vi "Write to Waveform Log Instance.vi"(6 "tf Modified?":bool, 7 "Wfm Index":i32, 8 "error in (no error)":errorcluster, 9 "Data":dbl[](array[numeric]), 10 "Waveform Data":T5, 11 "Log Instance in":T1) -> (0 "error out":errorcluster, 3 "Log Instance out":T1)   [LabVIEW 2015, in "Waveform Log.lvclass"]
uses:
  Waveform Log.lvclass
  Log Instance.ctl
  Logs/Segmented Logs/Segmented Log/Segmented Log.lvclass
  Log Instance Waveform.ctl
  Waveform Information.ctl
  Waveform Data Type.ctl
  Waveform Log Wfm Meta Data.ctl
  Logs/Segmented Logs/Segmented Log/Segmented Log Waveform Meta Data.ctl
  Logs/Segmented Logs/Segmented Log/Segmented Log.lvclass/Segmented Log.ctl
  Log File Specifications/Log File Specification/Log File Specification.lvclass/Log File Specification.ctl
  Log File Specifications/Waveform TDMS Log File Specification/Waveform TDMS Log File Specification.lvclass/Waveform TDMS Log File Specification.ctl
  Logs/Log Files/Log File/Log File.lvclass/Log File.ctl
  Logs/Log Files/TDMS Log File/TDMS Log File.lvclass/TDMS Log File.ctl
  Logs/Log Files/Text Log File/Text Log File.lvclass/Text Log File.ctl
  Logs/Segmented Logs/Footprint Segmented Log/Footprint Segmented Log.lvclass/Footprint Segmented Log.ctl
  Logs/Segmented Logs/Time Segmented Log/Time Segmented Log.lvclass/Time Segmented Log.ctl
  Log File Specifications/Log File Specification/Get Log Specification Type.vi
  Log File Specifications/Waveform TDMS Log File Specification/Get Current Group.vi
  Logs/Log Files/Log File/Get Log File Type.vi
  Logs/Log Files/Log File/Write Channel to Log File.vi
  Logs/Log Files/TDMS Log File/Set TDMS Channel Property.vi
  Logs/Log Files/TDMS Log File/Copy Channel Properties.vi
  Logs/Segmented Logs/Segmented Log/Check Close File.vi
  Logs/Segmented Logs/Segmented Log/Check Open File.vi
  Logs/Log Files/TDMS Log File/Write Channel to TDMS Log File.vi
  Logs/Log Files/Text Log File/Write Channel to Text Log File.vi
  Logs/Segmented Logs/Segmented Log/Close Log File Instance.vi
  Logs/Segmented Logs/Segmented Log/Segment Log File.vi
  Logs/Segmented Logs/Segmented Log/Open Log File Instance.vi
  Logs/Log Files/Log File/Close Log File.vi
  Logs/Segmented Logs/Segmented Log/Make File Read-Only.vi
  Logs/Segmented Logs/Segmented Log/On Segmented Log Complete.vi
  Logs/Segmented Logs/Segmented Log/On File Close.vi
  Logs/Segmented Logs/Footprint Segmented Log/Segment Log File (Footprint).vi
  Logs/Segmented Logs/Time Segmented Log/Segment Log File (Time).vi
  Log File Specifications/Log File Specification/Open Log File.vi
  Log File Specifications/Log File Specification/Set Path Tag.vi
  Logs/Segmented Logs/Segmented Log/On File Open.vi
  Log File Specifications/Log File Specification/Set Filename Offset.vi
  Logs/Log Files/TDMS Log File/Close TDMS Log File.vi
  Logs/Log Files/Text Log File/Close Text Log File.vi
  Logs/Segmented Logs/Segmented Log/Get Current Log File Instance.vi
  Logs/Log Files/Log File/Get File Size.vi
  Logs/Log Files/Log File/Get Start Time.vi
  Log File Specifications/Log File Specification/Build File Path.vi
  Log File Specifications/Log File Specification/Resolve File Conflicts.vi
  Shared/Utility/Format File Path for Linux.vi
  <vilib>/Utility/error.llb/Error Cluster From Error Code.vi
  Log File Specifications/Log File Specification/Initialize Log File.vi
  <vilib>/Utility/libraryn.llb/Create Directory Recursive.vi
  <vilib>/Utility/libraryn.llb/Check if File or Folder Exists.vi
  <vilib>/Utility/libraryn.llb/Get File Extension.vi
  Logs/Log Files/Text Log File/Text Log File.lvclass
  Logs/Log Files/TDMS Log File/TDMS Log File.lvclass
  Logs/Log Files/Log File/Log File.lvclass
  Logs/Segmented Logs/Time Segmented Log/Time Segmented Log.lvclass
  Logs/Segmented Logs/Footprint Segmented Log/Footprint Segmented Log.lvclass
  Log File Specifications/Waveform TDMS Log File Specification/Waveform TDMS Log File Specification.lvclass
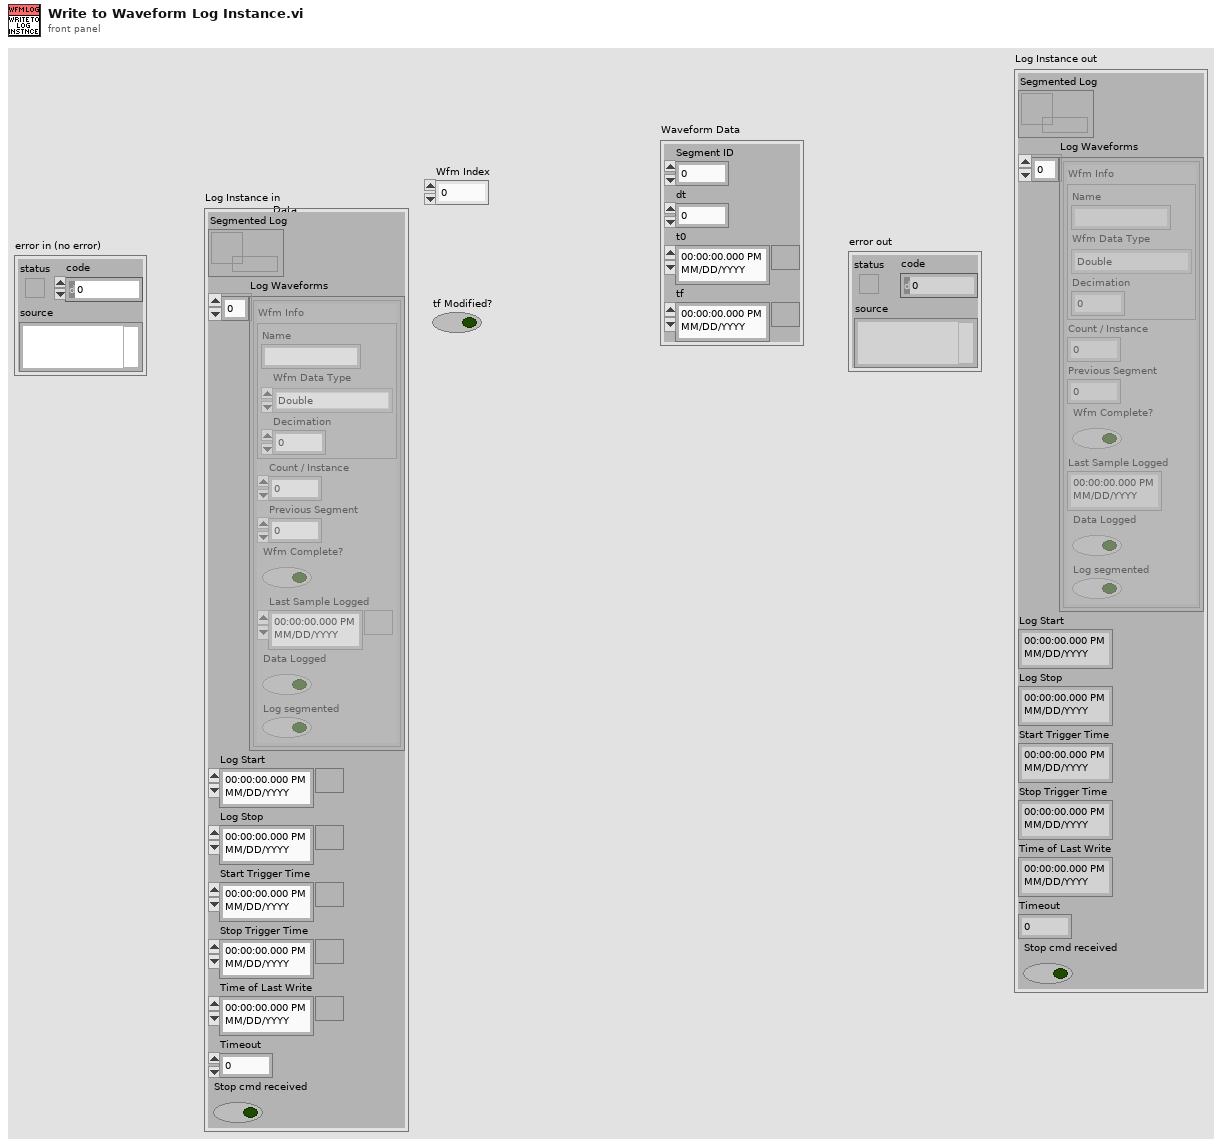
[diagram p1: front panel]
types:
  T1 = typedef "Waveform Log.lvclass/Log Instance.ctl" = cluster{"Segmented Log":refnum<data-value>, "Log Waveforms":T2[], "Log Start":timestamp, "Log Stop":timestamp, "Start Trigger Time":timestamp, "Stop Trigger Time":timestamp, "Time of Last Write":timestamp, "Timeout":dbl, "Stop cmd received":bool}
  T2 = typedef "Waveform Log.lvclass/Log Instance Waveform.ctl" = cluster{"Wfm Info":T3, "Count / Instance":i32, "Previous Segment":u64, "Wfm Complete?":bool, "Last Sample Logged":timestamp, "Data Logged":bool, "Log segmented":bool}
  T3 = typedef "Waveform Log.lvclass/Waveform Information.ctl" = cluster{"Name":string, "Wfm Data Type":T4, "Decimation":u32}
  T4 = typedef "Waveform Log.lvclass/Waveform Data Type.ctl" = enum16{"Double", "ComplexDouble"}
  T5 = typedef "Waveform Log.lvclass/Waveform Log Wfm Meta Data.ctl" = cluster{"Segment ID":u64, "dt":dbl, "t0":timestamp, "tf":timestamp}
  T6 = typedef "Segmented Log.lvclass/Segmented Log Waveform Meta Data.ctl" = cluster{"New Wfm Instance?":bool, "Wfm Instance":i32, "dt":dbl, "t0":timestamp}
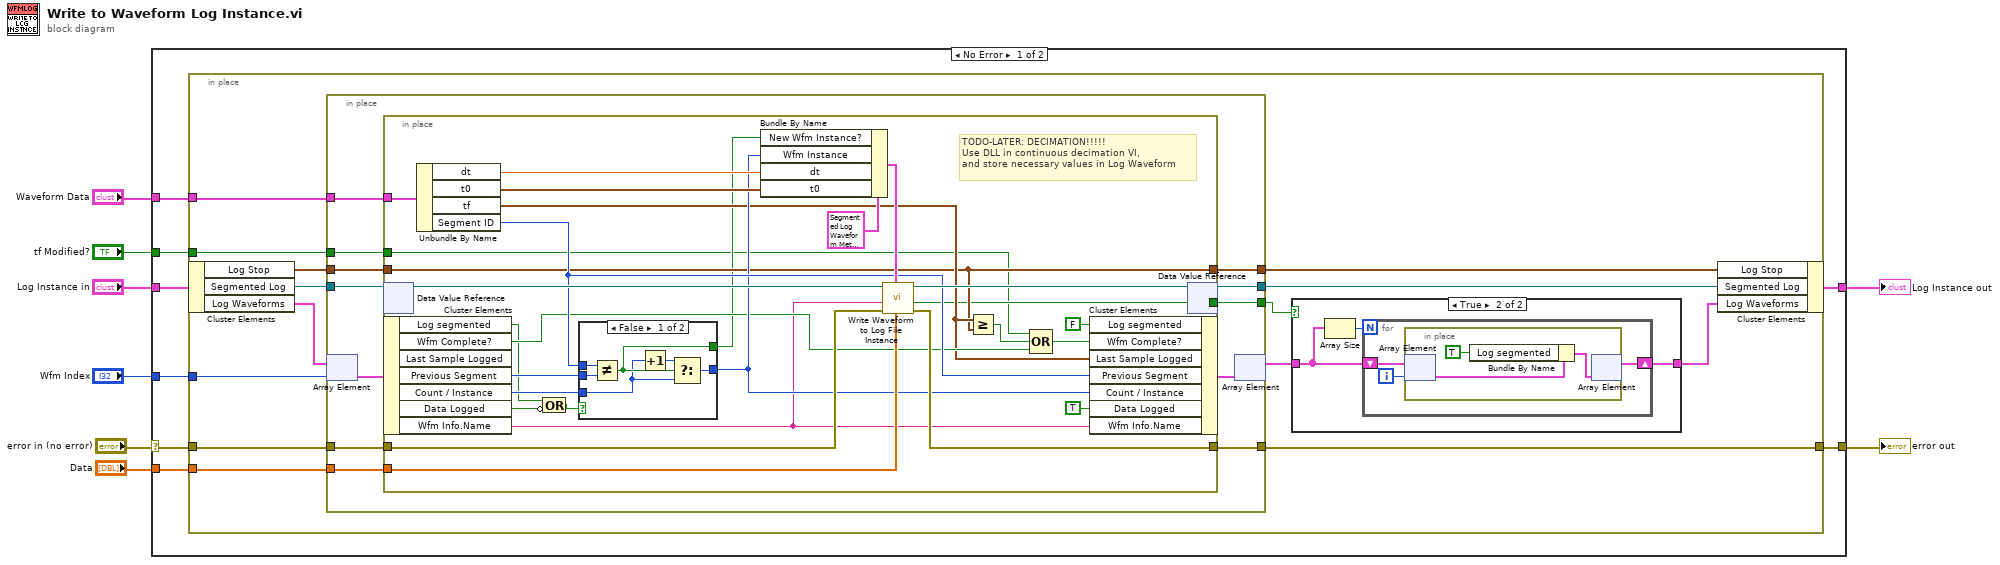
[diagram p0: block diagram]
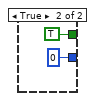
[diagram p3: hidden frame]
diagram:
  n1 = case shown="No Error" "error in (no error)" {
    selector: "error in (no error)" -> [w15 w90]
    tunnel: [w14 w90] -> w7
    tunnel: "Data" -> [w16 _]
    tunnel: "Log Instance in" -> [w13 w89]
    tunnel: "Wfm Index" -> [w12 _]
    tunnel: "Waveform Data" -> [w11 _]
    tunnel: [w10 w89] -> w2
    tunnel: "tf Modified?" -> [w9 _]
    frame No Error {
      n2 = in-place {
        in-place-border: w16 -> [w30]
        in-place-border: w15 -> [w29]
        in-place-border: [w17] -> w14
        in-place-border: w12 -> [w26]
        in-place-border: w11 -> [w25]
        in-place-border: w9 -> [w21]
        n3 = in-place-cluster #1(w13) -> ("Log Stop"=w23:timestamp, "Segmented Log"=w28:refnum<data-value>, "Log Waveforms"=w27:T2[])
        n4 = in-place {
          in-place-border: w30 -> [w52]
          in-place-border: w29 -> [w51]
          in-place-border: [w50] -> w17
          in-place-border: w28 -> [w49]
          in-place-border: w25 -> [w47]
          in-place-border: [w45] -> w24
          in-place-border: w23 -> [w44]
          in-place-border: [w43] -> w22
          in-place-border: [w42] -> w18
          in-place-border: w21 -> [w41]
          n5 = in-place-array #2(w27, w26) -> (w48:T2)
          n6 = in-place {
            in-place-border: w52 -> [w80]
            in-place-border: w51 -> [w79]
            in-place-border: [w78] -> w50
            in-place-border: w47 -> [w73]
            in-place-border: w44 -> [w63]
            in-place-border: [w63] -> w43
            in-place-border: [w56] -> w42
            in-place-border: w41 -> [w55]
            # "TODO-LATER: DECIMATION!!!!!\nUse DLL in continuous decimation VI,\nand store necessary values in Log Waveform"
            n7 = in-place-dvr #3(w49) -> (w76:refnum<class "Segmented Log.lvclass">)  [unwired: 1 out]
            n8 = in-place-cluster #4(w48) -> ("Log segmented"=w54:bool, "Wfm Complete?"=w66:bool, "Previous Segment"=w68:u64, "Count / Instance"=w67:i32, "Data Logged"=w58:bool, "Wfm Info.Name"=w60:string)  [unwired: 1 out]
            n9 = Unbundle By Name(w73) -> ("dt"=w72:dbl, "t0"=w71:timestamp, "tf"=w64:timestamp, "Segment ID"=w70:u64)
            n10 = Compound Arithmetic op=OR(w54, invert w58) -> (w57:bool)
            n11 = case shown="False" w57 {
              tunnel: w70 -> [w85 _]
              tunnel: [w84 0 ("Count / Instance")] -> w69
              tunnel: w68 -> [w83 _]
              tunnel: w67 -> [w81 _]
              tunnel: [w82 TRUE] -> w61
              frame False {
                n12 = Not Equal?(x=w85, y=w83) -> (x != y?=w82:bool)
                n13 = Increment(x=w81) -> (x+1=w86:i32)
                n14 = Select(t=w86, s=w82, f=w81) -> (s? t:f=w84:i32)
              }
              frame True {
              }
            }
            n15 = Bundle By Name(cluster=T6 {"New Wfm Instance?"=FALSE, "Wfm Instance"=0, "dt"=0.0, "t0"=timestamp(0 s since 1904-01-01)} ("Segmented Log Waveform Meta Data"), "New Wfm Instance?"=w61, "Wfm Instance"=w69, "dt"=w72, "t0"=w71) -> (w74:T6)
            n16 = call "Write Waveform to Log File Instance.vi"("Data"=w80, "Segmented Log Waveform Meta Data"=w74, "error in (no error)"=w79, "Channel Name in"=w60, "Segmented Log in"=w76) -> ("error out"=w78:errorcluster, "File Segmented"=w56:bool, "Segmented Log out"=w77:refnum<class "Segmented Log.lvclass">)  [unwired: 3 in, 1 out]
            n17 = Greater Or Equal?(x=w64, y=w63) -> (x >= y?=w62:bool)
            n18 = Compound Arithmetic op=OR(w55, w62, w66) -> (w65:bool)
            n19 = in-place-cluster #4("Log segmented"=FALSE, "Wfm Complete?"=w65, "Last Sample Logged"=w64, "Previous Segment"=w70, "Count / Instance"=w69, "Data Logged"=TRUE, "Wfm Info.Name"=w60) -> (w46:T2)
            n20 = in-place-dvr #3(w77) -> (w45:refnum<data-value>)  [unwired: 1 out]
          }
          n21 = in-place-array #2(w46) -> (w20:T2[])  [unwired: 1 out]
        }
        n22 = case shown="True" w18 {
          tunnel: w20 -> [w31 w33]
          tunnel: [w31 w32] -> w19
          frame False {
          }
          frame True {
            n23 = Array Size(array=w33) -> (size(s)=w34:i32)
            n24 = for {
              N: w34 -> [_]
              shift-right: [w35] -> w32
              shift-left: w33 -> [w37]
              i -> [w36]
              n25 = in-place {
                n26 = in-place-array #5(w37, w36) -> (w40:T2)
                n27 = Bundle By Name(cluster=w40, "Log segmented"=TRUE) -> (w38:T2)
                n28 = in-place-array #5(w38) -> (w35:T2[])  [unwired: 1 out]
              }
            }
          }
        }
        n29 = in-place-cluster #1("Log Stop"=w22, "Segmented Log"=w24, "Log Waveforms"=w19) -> (w10:T1)
      }
    }
    frame Error {
    }
  }
  "error out" <- w7
  "Log Instance out" <- w2
